vi "Transform.vi"(8 "error in (no error)":errorcluster caption="entrée d'erreur (pas d'erreur)", 10 "X":cluster{"Key":string[], "Value":i32[]}, 11 "DictVectorizer.lvclass":refnum<class "DictVectorizer.lvclass">) -> (0 "error out":errorcluster caption="sortie d'erreur", 2 "Data":T1, 3 "DictVectorizer.lvclass":refnum<class "DictVectorizer.lvclass">)   [LabVIEW 2020, in "DictVectorizer.lvclass"]
doc: "Learn a list of feature name -> indices mappings.\n\nReturns : \n\n- self"
uses:
  DictVectorizer.lvclass
  DictVectorizer.lvclass/DictVectorizer.ctl
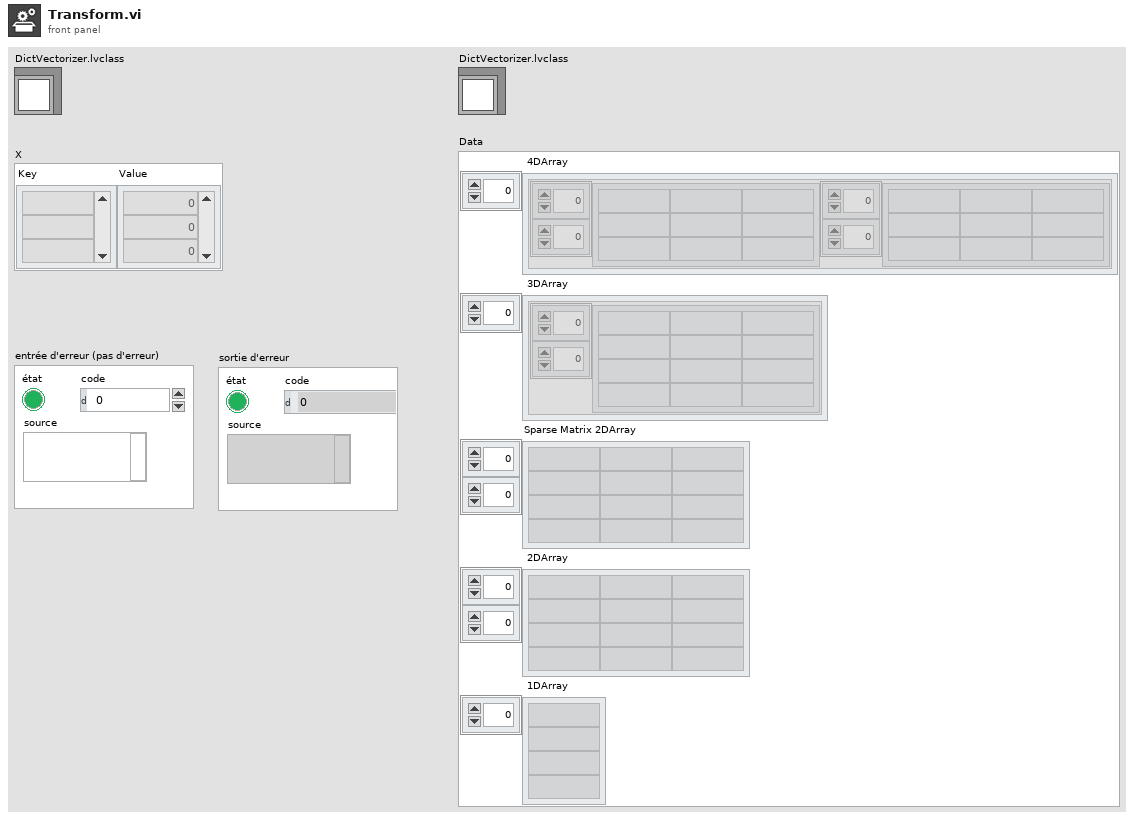
[diagram p1: front panel]
types:
  T1 = cluster{" 4DArray":cluster{"1":string[][], "2":string[][]}[], " 3DArray":cluster{"Tableau":string[][]}[], "Sparse Matrix 2DArray":string[][], " 2DArray":string[][], " 1DArray":string[]}
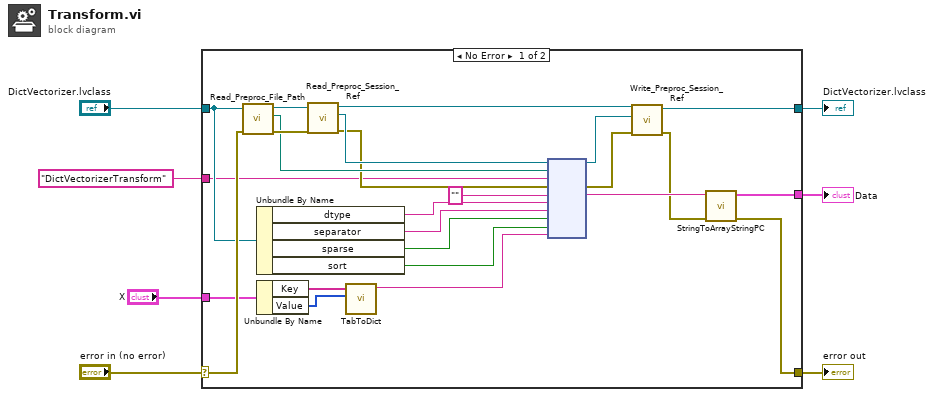
[diagram p0: block diagram]
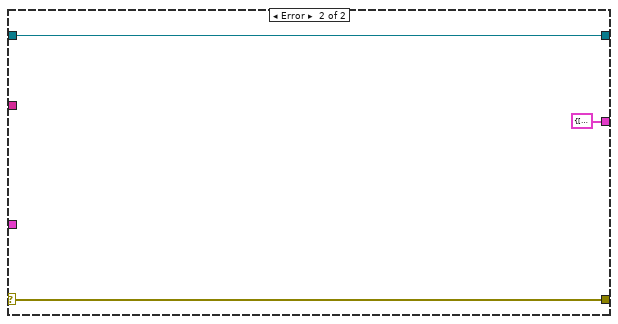
[diagram p2: hidden frame]
diagram:
  n1 = case shown="No Error" "error in (no error)" {
    selector: "error in (no error)" -> [w20 w35]
    tunnel: [w9 w35] -> w6
    tunnel: [w12 w34] -> w4
    tunnel: "DictVectorizer.lvclass" -> [w19 w34]
    tunnel: "DictVectorizerTransform" ("Fonction") -> [w18 _]
    tunnel: [w8 T1 {" 4DArray"=[], " 3DArray"=[], "Sparse Matrix 2DArray"=[], " 2DArray"=[], " 1DArray"=[]} ("Data")] -> w1
    tunnel: "X" -> [w15 _]
    frame No Error {
      n2 = call-dynamic "Read_Preproc_File_Path.vi"("error in (no error)"=w20, "Python in"=w19) -> ("error out"=w31:errorcluster, "File_Path"=w30:path, "Python out"=w32:refnum<class "DictVectorizer.lvclass">)  [unwired: 7 in]
      n3 = Unbundle By Name(w19) -> ("dtype"=w23:string, "separator"=w22:string, "sparse"=w21:bool, "sort"=w17:bool)
      n4 = Unbundle By Name(w15) -> ("Key"=w14:string[], "Value"=w16:i32[])
      n5 = call-dynamic "Read_Preproc_Session_Ref.vi"("error in (no error)"=w31, "Python in"=w32) -> ("error out"=w28:errorcluster, "Session_ref"=w29:refnum<k35>, "Python out"=w27:refnum<class "DictVectorizer.lvclass">)  [unwired: 7 in]
      n6 = call "TabToDict.vi"("Int Value"=w16, "String key"=w14) -> ("Dict with int value"=w13:string)  [unwired: 8 in, 1 out]
      n7 = node(w29, w30, w18, w28, "", w23, w22, w21, w17, w13) -> (w25:refnum<k35>, w26:errorcluster, w11:string)  [unwired: 5 in, 2 out]
      n8 = call-dynamic "Write_Preproc_Session_Ref.vi"("error in (no error)"=w26, "Session_ref"=w25, "Python in"=w27) -> ("error out"=w10:errorcluster, "Python out"=w12:refnum<class "DictVectorizer.lvclass">)  [unwired: 7 in]
      n9 = call "StringToArrayStringPC.vi"("sortie d'erreur"=w10, "Return value"=w11) -> ("sortie d'erreur"=w9:errorcluster, "Data"=w8:T1)  [unwired: 8 in]
    }
    frame Error {
    }
  }
  "error out" <- w6
  "DictVectorizer.lvclass" <- w4
  "Data" <- w1
